vi "ContRunMain.vi"(5 "line trig":bool=TRUE, 6 "Step Number":i32, 8 "error in":errorcluster, 9 "runs slider ref":refnum<vi>, 10 "image size":cluster{"xpixels":i32, "ypixels":i32}, 11 "Main Pulse In":T2) -> (0 "error out":errorcluster, 3 "readout":T1, 7 "Stop":bool)   [LabVIEW 2019]
uses:
  PulseControl.ctl
  Compiler/Params.ctl
  controls/GlobalExp.vi
  Global.lvlib
panel:
  out "DLL error code":u32
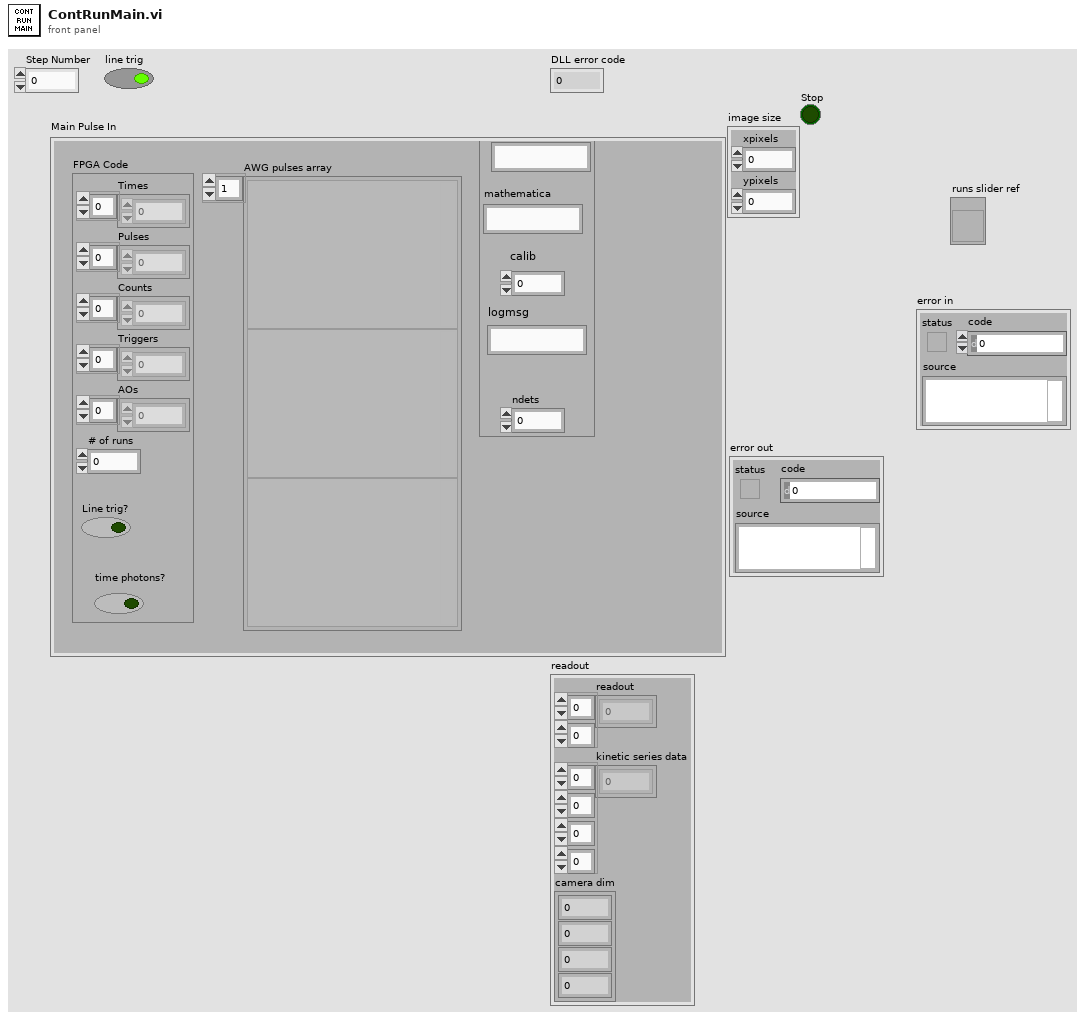
[diagram p1: front panel]
types:
  T1 = cluster{"readout":u32[][], "kinetic series data":i32[][][][], "camera dim":cluster{i32, i32, i32, i32}}
  T2 = typedef "PulseControl.ctl" = cluster{"FPGA Code":cluster{"Times":u32[], "Pulses":u64[], "Counts":u8[], "Triggers":u8[], "AOs":u8[], "# of runs":i32, "Line trig?":bool, "time photons?":bool}, "AWG pulses array":variant[], "Params":T3}
  T3 = typedef "Params.ctl" = cluster{"steps":i16, "runs":i16, "comment":string, "mathematica":string, "calib":i8, "logmsg":string, "ndets":i16}
  T4 = cluster{"Times":u32[], "Pulses":u64[], "Counts":u8[], "Triggers":u8[], "AOs":u8[], "# of runs":i32, "Line trig?":bool, "time photons?":bool}
  T5 = typedef "MasterExpControl.ctl" = cluster{"Main Steps":dbl, "Main Runs":dbl, "ExpStatus":enum16{"Innit", "Stop", "Idle", "MainRunning", "AuxRunning"}, "Main Current Step":dbl, "ExpNum":dbl, "NewData":bool, "date":string, "command":string, "Stop":bool, "Pause":bool, "Mathematica":string, "Main/Meta":bool, "UpdateMath":bool, "Camera":bool, "MetaExpOver":bool, "NextMetaExp":bool}
  T6 = cluster{"readout":i16[][], "kinetic series data":i32[][][][], "camera dim":cluster{i32, i32, i32, i32}}
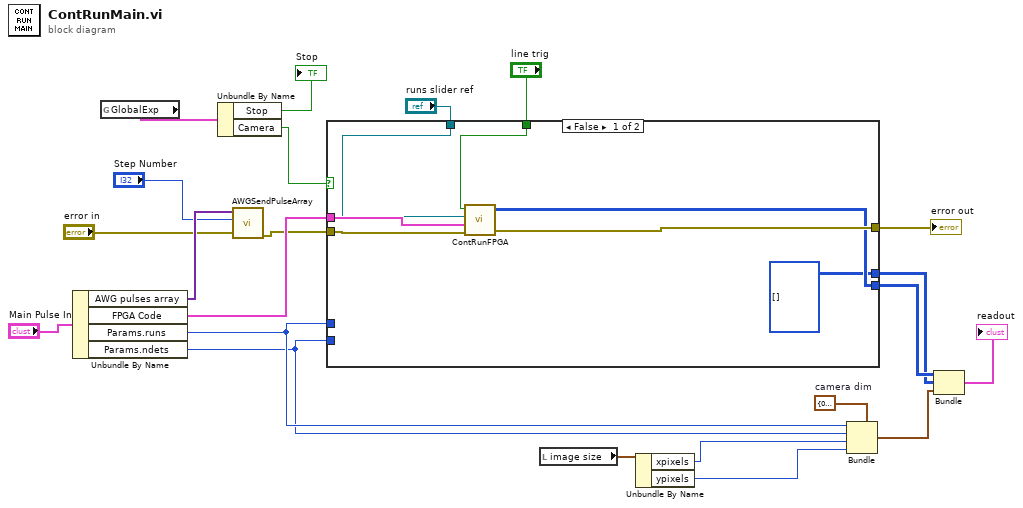
[diagram p0: block diagram]
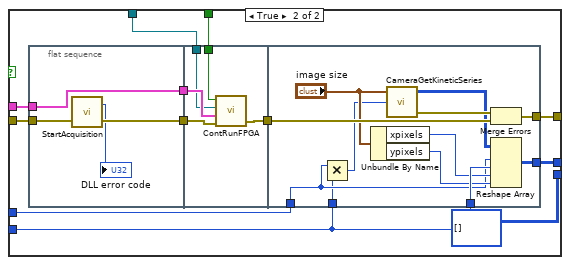
[diagram p2: hidden frame]
diagram:
  w17 = cluster{i32, i32, i32, i32} {0, 0, 0, 0}  # camera dim
  n1 = Unbundle By Name("Main Pulse In") -> ("AWG pulses array"=w5:variant[], "FPGA Code"=w21:T4, "Params.runs"=w15:i16, "Params.ndets"=w14:i16)
  n2 = global read "GlobalExp.vi" "GlobalExp"() -> (w9:T5)
  n3 = Unbundle By Name(w9) -> ("Stop"=→"Stop":bool, "Camera"=w7:bool)
  n4 = call "AWGSendPulseArray.vi"("error in (no error)"="error in", "Step Number"="Step Number", "AWG pulses array"=w5) -> ("error out"=w3:errorcluster)  [unwired: 8 in]
  n5 = case shown="False" w7 {
    tunnel: w21 -> [w29 w41]
    tunnel: [w26 i16[][] [] ("readout")] -> w19
    tunnel: w3 -> [w28 w40]
    tunnel: [w27 w39] -> w20
    tunnel: w15 -> [_ w35]
    tunnel: w14 -> [_ w32]
    tunnel: [i16[][][][] [] ("kinetic series data") w34] -> w18
    tunnel: "runs slider ref" -> [w24 w31]
    tunnel: "line trig" -> [w23 w30]
    frame False {
      n6 = call "ContRunFPGA.vi"("error in"=w28, "Cluster"=w29, "runs slider ref"=w24, "Line trig?"=w23) -> ("error out"=w27:errorcluster, "readout"=w26:i16[][])  [unwired: 1 out]
    }
    frame True {
      n7 = flat-sequence {
        tunnel: w40 -> [w44]
        tunnel: w41 -> [w45]
        tunnel: [w45] -> w38
        tunnel: [w43] -> w37
        tunnel: w38 -> [w50]
        tunnel: w37 -> [w49]
        tunnel: [w48] -> w36
        tunnel: w31 -> [w47]
        tunnel: w30 -> [w46]
        tunnel: [w60] -> w39
        tunnel: w36 -> [w61]
        tunnel: w35 -> [w52]
        tunnel: w32 -> [w58]
        tunnel: [w54] -> w34
        tunnel: w32 -> [w51]
        frame #0 {
          n8 = call <userlib>:"StartAcquisition.vi"("error in (no error)"=w44) -> ("error out"=w43:errorcluster, "DLL error code"=→"DLL error code":u32)  [unwired: 1 in]
        }
        frame #1 {
          n9 = call "ContRunFPGA.vi"("error in"=w49, "Cluster"=w50, "runs slider ref"=w47, "Line trig?"=w46) -> ("error out"=w48:errorcluster)  [unwired: 2 out]
        }
        frame #2 {
          n10 = Multiply(x=w52, y=w51) -> (x*y=w53:i16)
          n11 = Unbundle By Name("image size") -> ("xpixels"=w56:i32, "ypixels"=w55:i32)
          n12 = call "CameraGetKineticSeries.vi"("# of kinetics"=w53, "image size"="image size") -> ("error out"=w62:errorcluster, "kinetic series data"=w59:i32[][][])  [unwired: 2 in]
          n13 = Merge Errors(w62, w61) -> (w60:errorcluster)
          n14 = Reshape Array(w59, w52, w58, w56, w55) -> (w54:i32[][][][])
        }
      }
    }
  }
  "error out" <- w20
  n15 = local read "image size"() -> (w13:cluster{"xpixels":i32, "ypixels":i32})
  n16 = Unbundle By Name(w13) -> ("xpixels"=w12:i32, "ypixels"=w11:i32)
  n17 = Bundle(cluster=w17, w15, w14, w12, w11) -> (w16:cluster{i32, i32, i32, i32})
  n18 = Bundle("readout"=w19, "kinetic series data"=w18, "camera dim"=w16) -> (→"readout":T6)  [unwired: 1 in]
